vi "MatrixVg.vi"(3 "Time Stamp":timestamp, 6 "Play Button":bool, 8 "Custom Folder":string, 9 "Settings":T1={"Ring 3"=1, "Ring 2"=4, "Fixed Current mkA"=0.5, "If yes, the current is:"=enum."Radio Selection 1", "Ressitance measurements?"=TRUE, "Commute DC current?"=FALSE} {"Ring 3" items=["1 kOhm", "10 kOhm", "100 kOhm", "1 Mohm", "10 mOhm"]; "Ring 2" items=["1 kOhm", "10 kOhm", "100 kOhm", "1 Mohm", "10 MOhm"]}, 10 "Instruments":T2={"Oscillator"=TRUE, "Addr 1 lock-in"=TRUE, "Addr 1 lock-in oop"=TRUE, "Addr 2 lock-in"=FALSE, "Addr 2 lock-in oop"=FALSE, "Addr 3 lock-in"=FALSE, "Addr 3 lock-in oop"=FALSE, "Voltage (Vk1)"=FALSE, "Current (Ik1)"=TRUE, "Voltage (Vk2)"=FALSE, "Current (Ik2)"=FALSE, "Voltage (Vk3)"=FALSE, "Current (Ik3)"=FALSE, "Channel 1 (Vnano1)  "=FALSE, "Channel 2 (Vnano1b)"=FALSE, "Channel 1 (Vnano2)   "=FALSE, "Channel 2 (Vnano2b)"=FALSE, "Thermometer 1 (T1)"=TRUE, "Magnetic Field (B)"=TRUE, "Capacitance (C) and Loss (L)"=FALSE}, 11 "VgCluster":T3={"V1 (V)"=-1.0, "V2 (V)"=1.0, "Sweep rate, V/min"=1.0, "Time btw \npoints, sec"=1.0, "points at each Vg"=1, "Compliance, mkA"=0.05, "No-record rate, V/min"=30.0, "Full sweep?"=FALSE} {"No-record rate, V/min" min=0.0 max=1.0 step=0.01 format="%_4f"; "V2 (V)" min=-4.0 max=4.0 step=0.1 format="%.1f"; "Compliance, mkA" min=0.0 max=1.0 step=0.01 format="%.3f"; "Time btw \npoints, sec" format="%.2f"; "Sweep rate, V/min" min=0.0 max=1.0 step=0.01 format="%_4f"; "V1 (V)" min=-4.0 max=4.0 step=0.1 format="%.1f"}) -> ()   [LabVIEW 2017]
uses:
  <vilib>/Utility/file.llb/Read From Spreadsheet File (DBL).vi
panel:
  out "ArraySens 2":i8[](array[numeric])
  out "String":string
  out "Experiment ends at:":string
  out "Hours":dbl format="%.1f"
  out "Estimated time of experiment:":i16
  out "ArraySens":i8[](array[numeric])
  out "ArrayOsc":dbl[](array[numeric])
  out "# of configurations":i8
  out "Large Array":bool[][][](array[boolean])
  out "Contact configuration file (*.conf)":path
  # "hours"
  # "min.="
  # "Lock-in Amplifiers"
  # "Temperature"
  # "SourceMeters"
  # "Nanovoltmeters"
  # "Main"
  # "(not recommended, too slow)"
  # "Magnetic Field"
  # "Capacitance & Loss"
  # "(not recommended, too slow)"
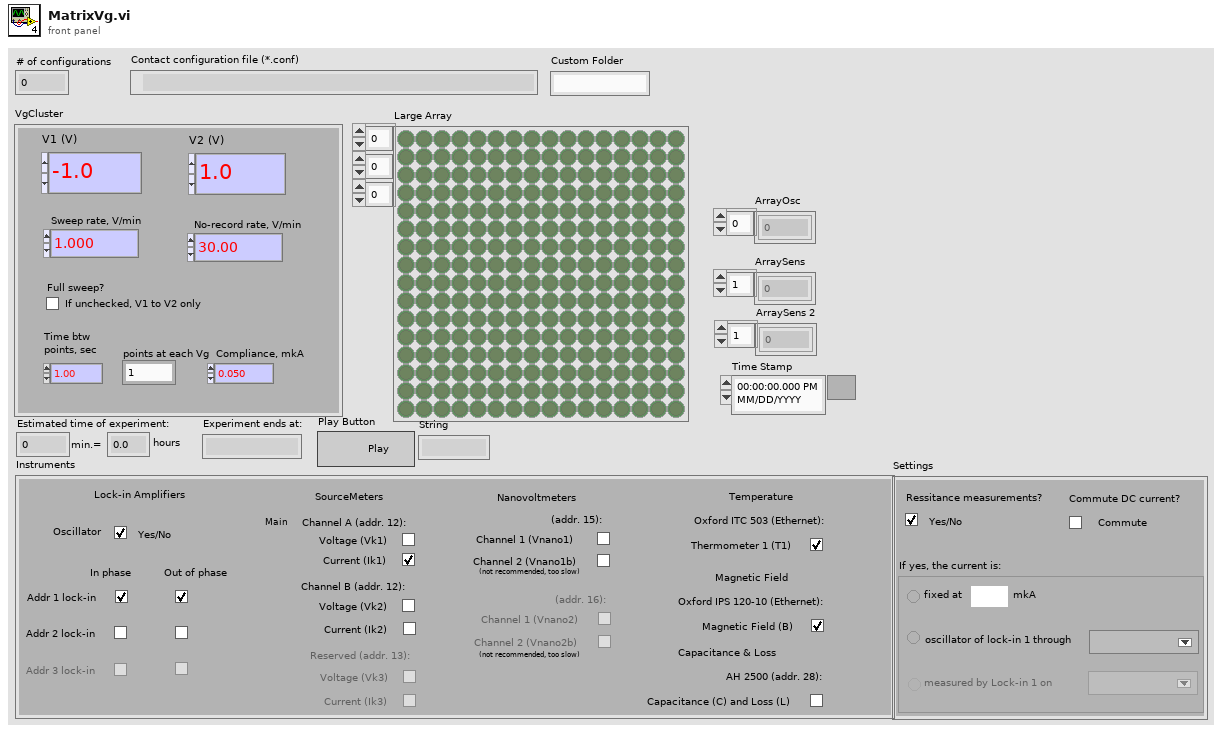
[diagram p1: front panel]
types:
  T1 = cluster{"Ring 3":u16, "Ring 2":u16, "Fixed Current mkA":dbl, "If yes, the current is:":enum32{"Radio Selection 1", "Radio Selection 2", "Radio Selection 3"}, "Ressitance measurements?":bool, "Commute DC current?":bool}
  T2 = cluster{"Oscillator":bool, "Addr 1 lock-in":bool, "Addr 1 lock-in oop":bool, "Addr 2 lock-in":bool, "Addr 2 lock-in oop":bool, "Addr 3 lock-in":bool, "Addr 3 lock-in oop":bool, "Voltage (Vk1)":bool, "Current (Ik1)":bool, "Voltage (Vk2)":bool, "Current (Ik2)":bool, "Voltage (Vk3)":bool, "Current (Ik3)":bool, "Channel 1 (Vnano1)  ":bool, "Channel 2 (Vnano1b)":bool, "Channel 1 (Vnano2)   ":bool, "Channel 2 (Vnano2b)":bool, "Thermometer 1 (T1)":bool, "Magnetic Field (B)":bool, "Capacitance (C) and Loss (L)":bool}
  T3 = cluster{"V1 (V)":dbl, "V2 (V)":dbl, "Sweep rate, V/min":dbl, "Time btw \npoints, sec":dbl, "points at each Vg":i32, "Compliance, mkA":dbl, "No-record rate, V/min":dbl, "Full sweep?":bool}
  T4 = cluster{"V2 (V)":dbl, "Sweep rate, V/min":dbl, "Time btw \npoints, sec":dbl, "points at each Vg":i32, "Compliance, mkA":dbl}
  T5 = cluster{"V1 (V)":dbl, "Sweep rate, V/min":dbl, "Time btw \npoints, sec":dbl, "points at each Vg":i32, "Compliance, mkA":dbl}
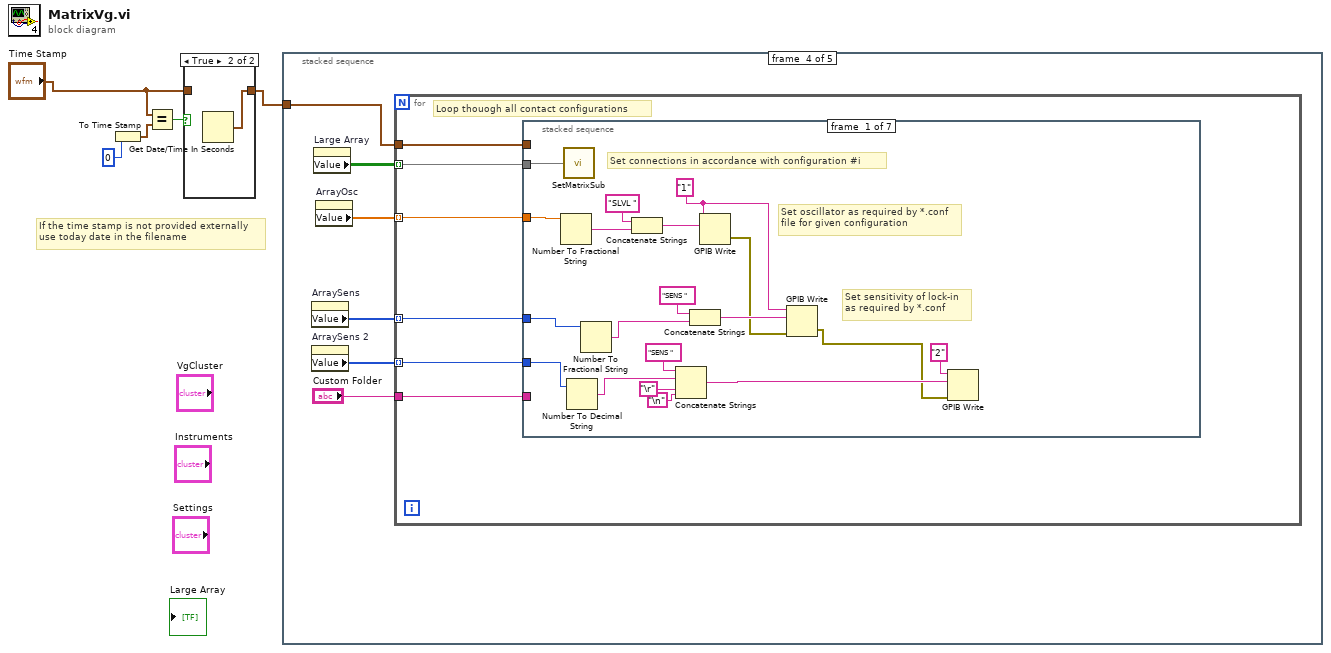
[diagram p0: block diagram]
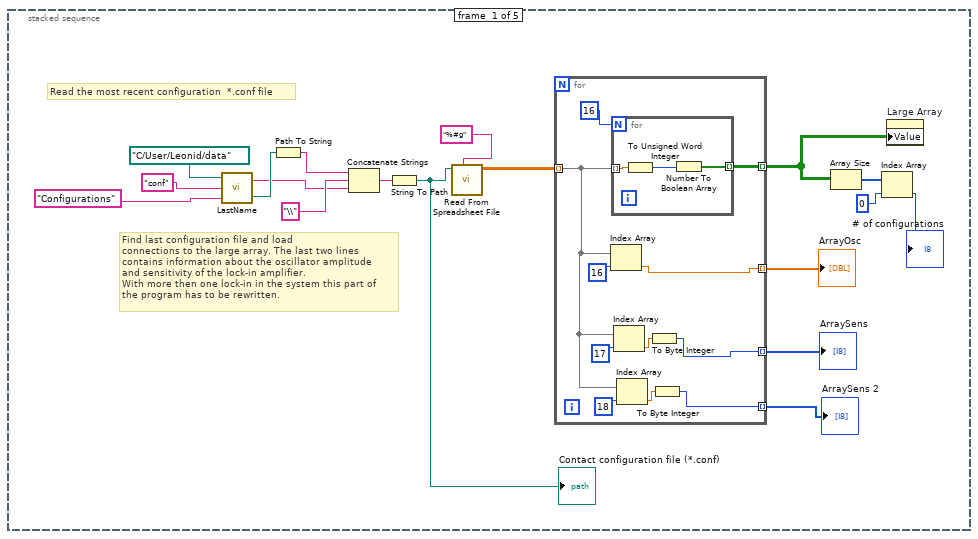
[diagram p3: hidden frame]
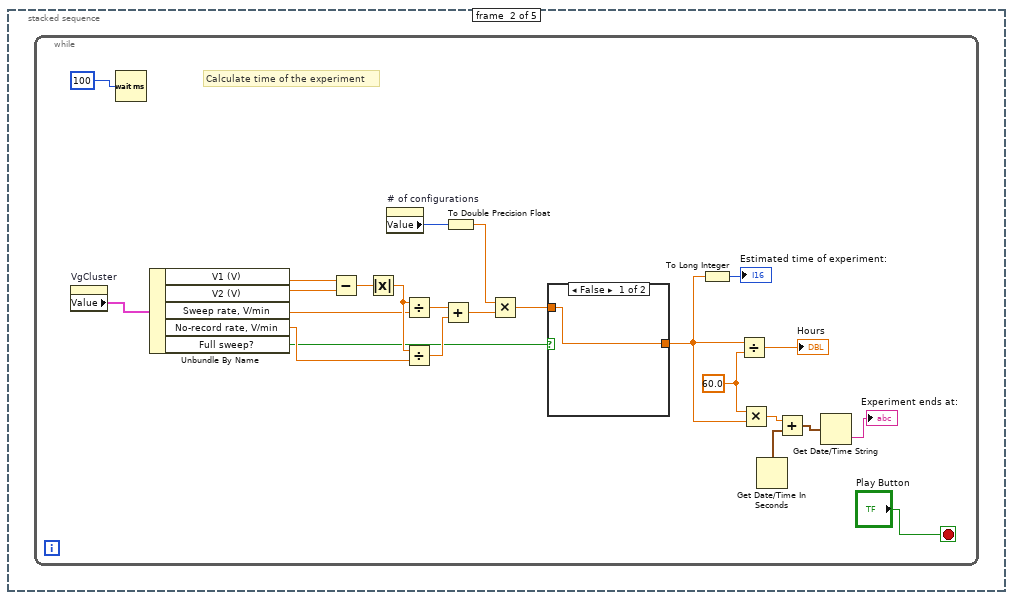
[diagram p4: hidden frame]
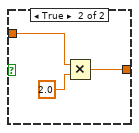
[diagram p5: hidden frame]
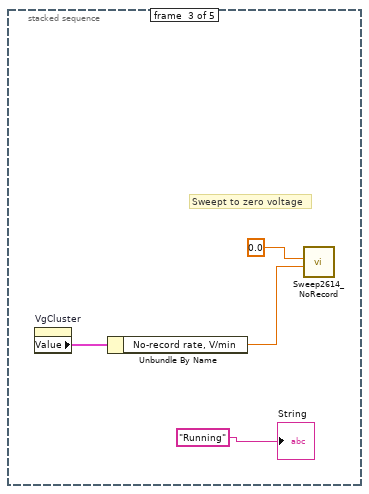
[diagram p6: hidden frame]
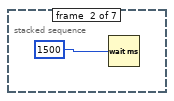
[diagram p7: hidden frame]
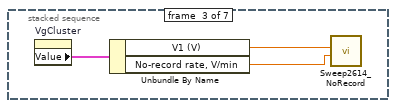
[diagram p8: hidden frame]
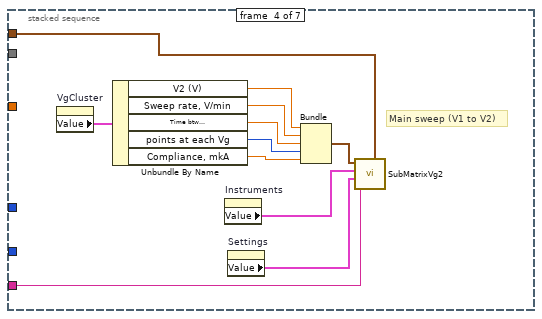
[diagram p9: hidden frame]
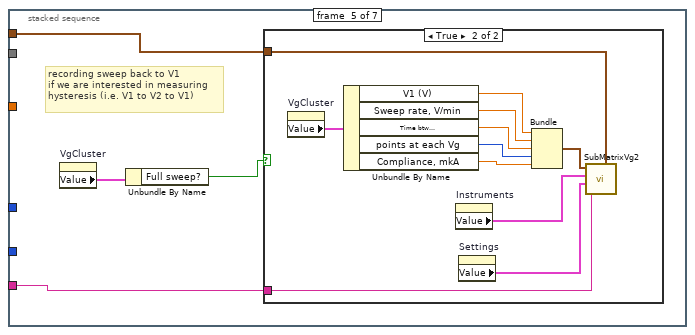
[diagram p10: hidden frame]
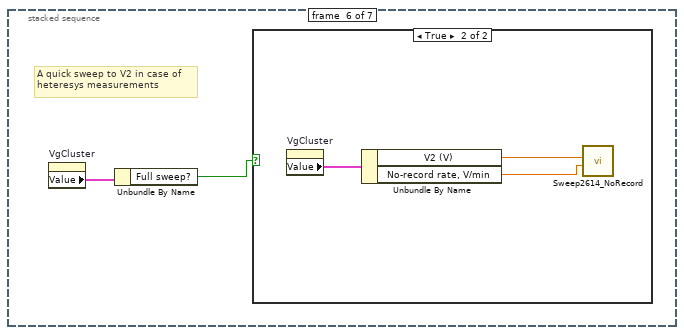
[diagram p12: hidden frame]
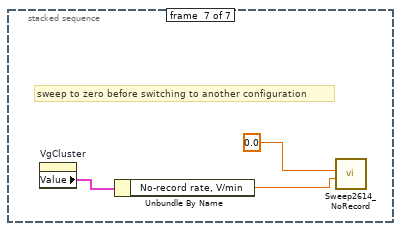
[diagram p14: hidden frame]
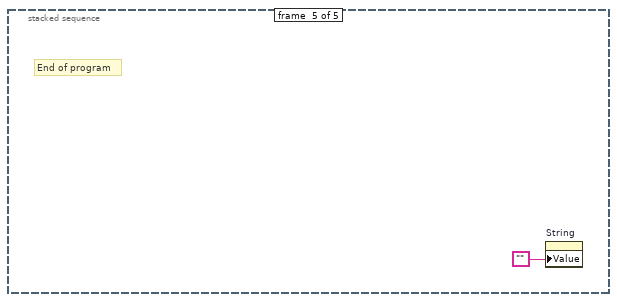
[diagram p15: hidden frame]
diagram:
  # "If the time stamp is not provided externally\nuse today date in the filename"
  n1 = To Time Stamp(1:0) -> (0:w4:timestamp)
  n2 = Equal?(x="Time Stamp", y=w4) -> (x = y?=w3:bool)
  n3 = case shown="True" w3 {
    tunnel: "Time Stamp" -> [w6 _]
    tunnel: [w6 w7] -> w1
    frame False {
    }
    frame True {
      n4 = Get Date/Time In Seconds() -> (seconds since 1Jan1904=w7:timestamp)
    }
  }
  n5 = stacked-sequence {
    tunnel: w1 -> [_ _ _ w73 _]
    frame #0 {
      # "Read the most recent configuration  *.conf file"
      # "Find last configuration file and load \nconnections to the large array. The last two lines \ncontains information about the oscillator amplitude\nand sensitivity of the lock-in amplifier.\nWith more then one lock-in in the system this part of \nthe program has to be rewritten."
      n6 = call "LastName.vi"("Custom Folder"="Configurations", "Extention"="conf", "User Data Folder"=path "C:/User/Leonid/data") -> ("created path"=w21:path, "String"=w20:string)
      n7 = Path To String(path=w21) -> (string=w25:string)
      n8 = Concatenate Strings(w25, "\\", w20) -> (w23:string)
      n9 = String To Path(string=w23) -> (path=w11:path)
      "Contact configuration file (*.conf)" <- w11
      n10 = call-poly <vilib>:"Read From Spreadsheet File.vi"("format (%.3f)"="%#g", "file path (dialog if empty)"=w11) -> ("all rows"=w16:dbl[][])  [unwired: 5 in, 4 out]
      n11 = for {
        tunnel: w16 -> [w27] mode=indexing
        tunnel: [w36] -> w13 mode=indexing
        tunnel: [w32] -> w10 mode=indexing
        tunnel: [w31] -> w9 mode=indexing
        tunnel: [w26] -> w8 mode=indexing
        n12 = Index Array(array=w27, index=16) -> (element=w32:dbl)
        n13 = for {
          N: 16 -> [_]
          tunnel: w27 -> [w39] mode=indexing
          tunnel: [w37] -> w36 mode=indexing
          n14 = To Unsigned Word Integer(number=w39) -> (unsigned 16bit integer=w38:u16)
          n15 = Number To Boolean Array(number=w38) -> (Boolean array=w37:bool[])
        }
        n16 = Index Array(array=w27, index=17) -> (element=w33:dbl)
        n17 = Index Array(array=w27, index=18) -> (element=w28:dbl)
        n18 = To Byte Integer(number=w33) -> (8bit integer=w31:i8)
        n19 = To Byte Integer(number=w28) -> (8bit integer=w26:i8)
      }
      "ArrayOsc" <- w10
      "ArraySens" <- w9
      "ArraySens 2" <- w8
      n20 = Array Size(array=w13) -> (size(s)=w15:i32[])
      n21 = Index Array(array=w15, index=0) -> (element=→"# of configurations":i32)
      n22 = property on="Large Array" class="Arr (strict)"("Value"=w13) -> ()  [unwired: 2 in, 2 out]
    }
    frame #1 {
      n23 = while {
        stop <- "Play Button" stop-if-true
        w42 = 60.0
        # "Calculate time of the experiment"
        n24 = property on="VgCluster" class="Clust (strict)"() -> ("Value"=w61:T3)  [unwired: 2 in, 2 out]
        n25 = Wait (ms)(milliseconds to wait=100) -> ()  [unwired: 1 out]
        n26 = Unbundle By Name(w61) -> ("V1 (V)"=w60:dbl, "V2 (V)"=w59:dbl, "Sweep rate, V/min"=w56:dbl, "No-record rate, V/min"=w55:dbl, "Full sweep?"=w49:bool)
        n27 = Subtract(x=w60, y=w59) -> (x-y=w58:dbl)
        n28 = Absolute Value(x=w58) -> (abs(x)=w57:dbl)
        n29 = property on="# of configurations" class="DigNum (strict)"() -> ("Value"=w51:i8)  [unwired: 2 in, 2 out]
        n30 = Divide(x=w57, y=w56) -> (x/y=w54:dbl)
        n31 = Divide(x=w57, y=w55) -> (x/y=w53:dbl)
        n32 = Add(x=w54, y=w53) -> (x+y=w52:dbl)
        n33 = To Double Precision Float(number=w51) -> (double precision float=w50:dbl)
        n34 = Multiply(x=w50, y=w52) -> (x*y=w48:dbl)
        n35 = case shown="False" w49 {
          tunnel: w48 -> [w64 w67]
          tunnel: [w64 w65] -> w41
          frame False {
          }
          frame True {
            n36 = Multiply(x=w67, y=2.0) -> (x*y=w65:dbl)
          }
        }
        n37 = To Long Integer(number=w41) -> (32bit integer=→"Estimated time of experiment:":i32)
        n38 = Divide(x=w41, y=w42) -> (x/y=→"Hours":dbl)
        n39 = Multiply(x=w42, y=w41) -> (x*y=w40:dbl)
        n40 = Get Date/Time In Seconds() -> (seconds since 1Jan1904=w46:timestamp)
        n41 = Add(x=w40, y=w46) -> (x+y=w45:timestamp)
        n42 = Get Date/Time String(seconds (now)=w45) -> (time string=→"Experiment ends at:":string)  [unwired: 2 in, 1 out]
      }
    }
    frame #2 {
      # "Sweept to zero voltage"
      n43 = property on="VgCluster" class="Clust (strict)"() -> ("Value"=w70:T3)  [unwired: 2 in, 2 out]
      n44 = Unbundle By Name(w70) -> ("No-record rate, V/min"=w69:dbl)
      n45 = call "Sweep2614_NoRecord.vi"("Rate (V/min)"=w69, "Vfinal (V)"=0.0) -> ()  [unwired: 2 in, 1 out]
      "String" <- "Running"
    }
    frame #3 {
      n46 = property on="ArraySens" class="Arr (strict)"() -> ("Value"=w75:i8[])  [unwired: 2 in, 2 out]
      n47 = property on="ArraySens 2" class="Arr (strict)"() -> ("Value"=w72:i8[])  [unwired: 2 in, 2 out]
      n48 = property on="Large Array" class="Arr (strict)"() -> ("Value"=w77:bool[][][])  [unwired: 2 in, 2 out]
      n49 = property on="ArrayOsc" class="Arr (strict)"() -> ("Value"=w76:dbl[])  [unwired: 2 in, 2 out]
      n50 = for {
        tunnel: w77 -> [w83] mode=indexing
        tunnel: w76 -> [w82] mode=indexing
        tunnel: w75 -> [w81] mode=indexing
        tunnel: "Custom Folder" -> [w80]
        tunnel: w73 -> [w79]
        tunnel: w72 -> [w78] mode=indexing
        # "Loop thouogh all contact configurations"
        n51 = stacked-sequence {
          tunnel: w83 -> [w102 _ _ _ _ _ _]
          tunnel: w82 -> [w98 _ _ _ _ _ _]
          tunnel: w81 -> [w93 _ _ _ _ _ _]
          tunnel: w80 -> [_ _ _ w117 w121 _ _]
          tunnel: w79 -> [_ _ _ w116 w120 _ _]
          tunnel: w78 -> [w88 _ _ _ _ _ _]
          frame #0 {
            w94 = "1"
            # "Set sensitivity of lock-in\nas required by *.conf"
            # "Set oscillator as required by *.conf\nfile for given configuration"
            # "Set connections in accordance with configuration #i"
            n52 = Number To Fractional String(number=w98) -> (F-format string=w101:string)  [unwired: 3 in]
            n53 = call "SetMatrixSub.vi"("Array"=w102) -> ()  [unwired: 1 in]
            n54 = Number To Decimal String(number=w88) -> (decimal integer string=w91:string)  [unwired: 1 in]
            n55 = Number To Fractional String(number=w93) -> (F-format string=w97:string)  [unwired: 3 in]
            n56 = Concatenate Strings("SLVL ", w101) -> (w100:string)
            n57 = Concatenate Strings("SENS ", w91, "\r", "\n") -> (w90:string)
            n58 = Concatenate Strings("SENS ", w97) -> (w96:string)
            n59 = GPIB Write(0:w94, 1:w100) -> (6:w92:errorcluster)  [unwired: 3 in, 1 out]
            n60 = GPIB Write(0:w94, 1:w96, 3:w92) -> (6:w85:errorcluster)  [unwired: 2 in, 1 out]
            n61 = GPIB Write(0:"2", 1:w90, 3:w85) -> ()  [unwired: 2 in, 2 out]
          }
          frame #1 {
            n62 = Wait (ms)(milliseconds to wait=1500) -> ()  [unwired: 1 out]
          }
          frame #2 {
            n63 = property on="VgCluster" class="Clust (strict)"() -> ("Value"=w106:T3)  [unwired: 2 in, 2 out]
            n64 = Unbundle By Name(w106) -> ("V1 (V)"=w105:dbl, "No-record rate, V/min"=w104:dbl)
            n65 = call "Sweep2614_NoRecord.vi"("Rate (V/min)"=w104, "Vfinal (V)"=w105) -> ()  [unwired: 2 in, 1 out]
          }
          frame #3 {
            # "Main sweep (V1 to V2)"
            n66 = property on="VgCluster" class="Clust (strict)"() -> ("Value"=w115:T3)  [unwired: 2 in, 2 out]
            n67 = Unbundle By Name(w115) -> ("V2 (V)"=w114:dbl, "Sweep rate, V/min"=w113:dbl, "Time btw \npoints, sec"=w112:dbl, "points at each Vg"=w111:i32, "Compliance, mkA"=w110:dbl)
            n68 = property on="Instruments" class="Clust (strict)"() -> ("Value"=w108:T2)  [unwired: 2 in, 2 out]
            n69 = property on="Settings" class="Clust (strict)"() -> ("Value"=w107:T1)  [unwired: 2 in, 2 out]
            n70 = Bundle("V2 (V)"=w114, "Sweep rate, V/min"=w113, "Time btw \npoints, sec"=w112, "points at each Vg"=w111, "Compliance, mkA"=w110) -> (w109:T4)  [unwired: 1 in]
            n71 = call "SubMatrixVg2.vi"("VgCluster"=w109, "Instruments"=w108, "Settings"=w107, "Custom Folder"=w117, "Time Stamp"=w116) -> ()  [unwired: 5 in]
          }
          frame #4 {
            # "recording sweep back to V1\nif we are interested in measuring \nhysteresis (i.e. V1 to V2 to V1)"
            n72 = property on="VgCluster" class="Clust (strict)"() -> ("Value"=w119:T3)  [unwired: 2 in, 2 out]
            n73 = Unbundle By Name(w119) -> ("Full sweep?"=w118:bool)
            n74 = case shown="True" w118 {
              tunnel: w121 -> [_ w132]
              tunnel: w120 -> [_ w131]
              frame False {
              }
              frame True {
                n75 = property on="VgCluster" class="Clust (strict)"() -> ("Value"=w130:T3)  [unwired: 2 in, 2 out]
                n76 = Unbundle By Name(w130) -> ("V1 (V)"=w129:dbl, "Sweep rate, V/min"=w128:dbl, "Time btw \npoints, sec"=w127:dbl, "points at each Vg"=w126:i32, "Compliance, mkA"=w125:dbl)
                n77 = property on="Instruments" class="Clust (strict)"() -> ("Value"=w123:T2)  [unwired: 2 in, 2 out]
                n78 = property on="Settings" class="Clust (strict)"() -> ("Value"=w122:T1)  [unwired: 2 in, 2 out]
                n79 = Bundle("V1 (V)"=w129, "Sweep rate, V/min"=w128, "Time btw \npoints, sec"=w127, "points at each Vg"=w126, "Compliance, mkA"=w125) -> (w124:T5)  [unwired: 1 in]
                n80 = call "SubMatrixVg2.vi"("VgCluster"=w124, "Instruments"=w123, "Settings"=w122, "Custom Folder"=w132, "Time Stamp"=w131) -> ()  [unwired: 5 in]
              }
            }
          }
          frame #5 {
            # "A quick sweep to V2 in case of\nheteresys measurements"
            n81 = property on="VgCluster" class="Clust (strict)"() -> ("Value"=w134:T3)  [unwired: 2 in, 2 out]
            n82 = Unbundle By Name(w134) -> ("Full sweep?"=w133:bool)
            n83 = case shown="True" w133 {
              frame False {
              }
              frame True {
                n84 = property on="VgCluster" class="Clust (strict)"() -> ("Value"=w137:T3)  [unwired: 2 in, 2 out]
                n85 = Unbundle By Name(w137) -> ("V2 (V)"=w136:dbl, "No-record rate, V/min"=w135:dbl)
                n86 = call "Sweep2614_NoRecord.vi"("Rate (V/min)"=w135, "Vfinal (V)"=w136) -> ()  [unwired: 2 in, 1 out]
              }
            }
          }
          frame #6 {
            # "sweep to zero before switching to another configuration"
            n87 = property on="VgCluster" class="Clust (strict)"() -> ("Value"=w140:T3)  [unwired: 2 in, 2 out]
            n88 = Unbundle By Name(w140) -> ("No-record rate, V/min"=w139:dbl)
            n89 = call "Sweep2614_NoRecord.vi"("Rate (V/min)"=w139, "Vfinal (V)"=0.0) -> ()  [unwired: 2 in, 1 out]
          }
        }
      }
    }
    frame #4 {
      # "End of program"
      n90 = property on="String" class="Str"("Value"="") -> ()  [unwired: 2 in, 2 out]
    }
  }
